vi "Register gRPC Methods.vi"(8 "error in (no error)":errorcluster, 11 "Template Server in":refnum<class "PluginLoader.lvclass">) -> (0 "error out":errorcluster, 3 "Template Server out":refnum<class "PluginLoader.lvclass">)   [LabVIEW 2021, in "CIF_PluginLoader_server.lvlib" / "PluginLoader.lvclass"]
uses:
  PluginLoader.lvclass
  typeDefs/Server Internal UEs.ctl
  typeDefs/Server Internal Message.ctl
  typeDefs/Server gRPC UEs.ctl
  <vilib>/gRPC/LabVIEW gRPC Library/Server API/typeDefs/gRPCId Cluster.ctl
  <vilib>/gRPC/LabVIEW gRPC Library/Shared/grpcId.ctl
  PluginLoader.lvclass/PluginLoader.ctl
  <vilib>/gRPC/LabVIEW gRPC Library/grpc-lvsupport-release.lvlib
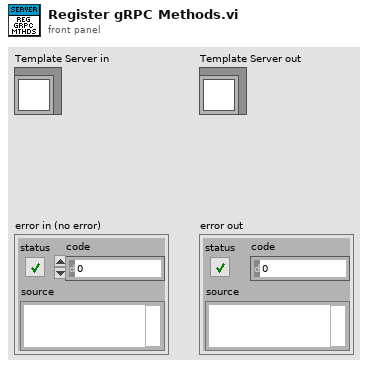
[diagram p1: front panel]
types:
  T1 = typedef "CIF_PluginLoader_server.lvlib/PluginLoader.lvclass/Server gRPC UEs.ctl" = cluster{"PluginLoader LoadPlugin gRPC UE":refnum<user-event>, "PluginLoader AbortPlugin gRPC UE":refnum<user-event>, "PluginLoader Destroy gRPC UE":refnum<user-event>, "PluginLoader Ping gRPC UE":refnum<user-event>, "PluginLoader Discover gRPC UE":refnum<user-event>}
  T2 = typedef "CIF_PluginLoader_server.lvlib/PluginLoader.lvclass/Server Internal UEs.ctl" = cluster{"PluginLoader LoadPlugin Internal UE":refnum<user-event>, "PluginLoader AbortPlugin Internal UE":refnum<user-event>, "PluginLoader Destroy Internal UE":refnum<user-event>, "PluginLoader Ping Internal UE":refnum<user-event>, "PluginLoader Discover Internal UE":refnum<user-event>}
  T3 = typedef "grpc-lvsupport-release.lvlib/grpcId.ctl" = u64
  T4 = typedef "CIF_PluginLoader_server.lvlib/PluginLoader.lvclass/Server Internal Message UE.ctl" = refnum<user-event>
  T5 = typedef "grpc-lvsupport-release.lvlib/gRPCId Cluster UE.ctl" = refnum<user-event>
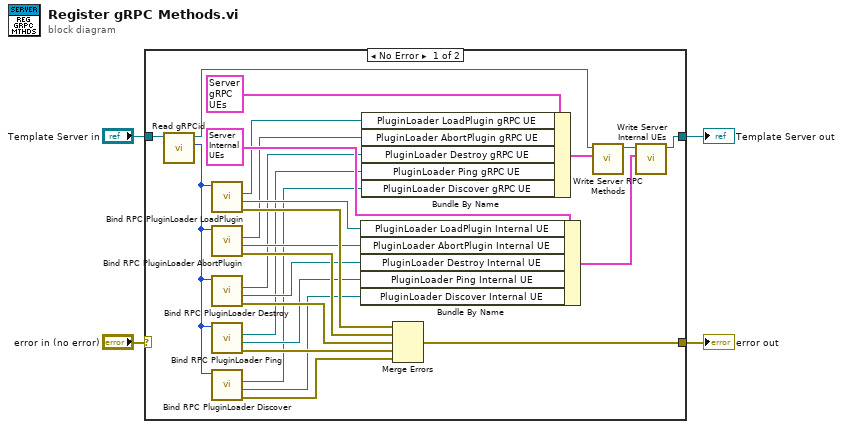
[diagram p0: block diagram]
diagram:
  n1 = case shown="No Error" "error in (no error)" {
    selector: "error in (no error)" -> [_ w30]
    tunnel: "Template Server in" -> [w21 w31]
    tunnel: [w29 w30] -> w3
    tunnel: [w28 w31] -> w2
    frame No Error {
      n2 = call-dynamic "Read gRPCid.vi"("iService in"=w21) -> ("gRPCid"=w20:T3, "iService out"=w22:refnum<class "PluginLoader.lvclass">)  [unwired: 8 in, 1 out]
      n3 = call "Bind RPC PluginLoader LoadPlugin.vi"("gRPCid server in"=w20) -> ("error out"=w19:errorcluster, "PluginLoader LoadPlugin Internal UE"=w17:T4, "PluginLoader LoadPlugin gRPC UE"=w18:T5)  [unwired: 7 in, 1 out]
      n4 = call "Bind RPC PluginLoader AbortPlugin.vi"("gRPCid server in"=w20) -> ("error out"=w16:errorcluster, "PluginLoader AbortPlugin Internal UE"=w14:T4, "PluginLoader AbortPlugin gRPC UE"=w15:T5)  [unwired: 7 in, 1 out]
      n5 = call "Bind RPC PluginLoader Destroy.vi"("gRPCid server in"=w20) -> ("error out"=w13:errorcluster, "PluginLoader Destroy Internal UE"=w12:T4, "PluginLoader Destroy gRPC UE"=w11:T5)  [unwired: 7 in, 1 out]
      n6 = call "Bind RPC PluginLoader Ping.vi"("gRPCid server in"=w20) -> ("error out"=w10:errorcluster, "PluginLoader Ping Internal UE"=w8:T4, "PluginLoader Ping gRPC UE"=w9:T5)  [unwired: 7 in, 1 out]
      n7 = call "Bind RPC PluginLoader Discover.vi"("gRPCid server in"=w20) -> ("error out"=w7:errorcluster, "PluginLoader Discover Internal UE"=w5:T4, "PluginLoader Discover gRPC UE"=w6:T5)  [unwired: 7 in, 1 out]
      n8 = Bundle By Name ("Bundle Internal UEs")(cluster=T2 {"PluginLoader LoadPlugin Internal UE"=refnum, "PluginLoader AbortPlugin Internal UE"=refnum, "PluginLoader Destroy Internal UE"=refnum, "PluginLoader Ping Internal UE"=refnum, "PluginLoader Discover Internal UE"=refnum} ("Server Internal UEs"), "PluginLoader LoadPlugin Internal UE"=w17, "PluginLoader AbortPlugin Internal UE"=w14, "PluginLoader Destroy Internal UE"=w12, "PluginLoader Ping Internal UE"=w8, "PluginLoader Discover Internal UE"=w5) -> (w27:T2)
      n9 = Bundle By Name ("Bundle gRPC UEs")(cluster=T1 {"PluginLoader LoadPlugin gRPC UE"=refnum, "PluginLoader AbortPlugin gRPC UE"=refnum, "PluginLoader Destroy gRPC UE"=refnum, "PluginLoader Ping gRPC UE"=refnum, "PluginLoader Discover gRPC UE"=refnum} ("gRPC Server Method Events"), "PluginLoader LoadPlugin gRPC UE"=w18, "PluginLoader AbortPlugin gRPC UE"=w15, "PluginLoader Destroy gRPC UE"=w11, "PluginLoader Ping gRPC UE"=w9, "PluginLoader Discover gRPC UE"=w6) -> (w24:T1)
      n10 = Merge Errors(w19, w16, w13, w10, w7) -> (w29:errorcluster)
      n11 = call "Write Server RPC Methods.vi"("Server RPC Methods"=w24, "SignalGeneratorService in"=w22) -> ("SignalGeneratorService out"=w25:refnum<class "PluginLoader.lvclass">)  [unwired: 8 in, 1 out]
      n12 = call "Write Server Internal UEs.vi"("Server Internal UEs"=w27, "SignalGeneratorService in"=w25) -> ("SignalGeneratorService out"=w28:refnum<class "PluginLoader.lvclass">)  [unwired: 8 in, 1 out]
    }
    frame Error {
    }
  }
  "error out" <- w3
  "Template Server out" <- w2
